vi "DN4_2Darray2DDT.vi"(3 "rate":dbl, 4 "StartTime":timestamp, 5 "2D Array":dbl[][](array[numeric])) -> (1 "Dynamic Data Type":dynamicdata(graph), 2 "EndTime":timestamp)   [LabVIEW 2009]
uses:
  Instance           1 19Saved   2Darray2DDT .vi
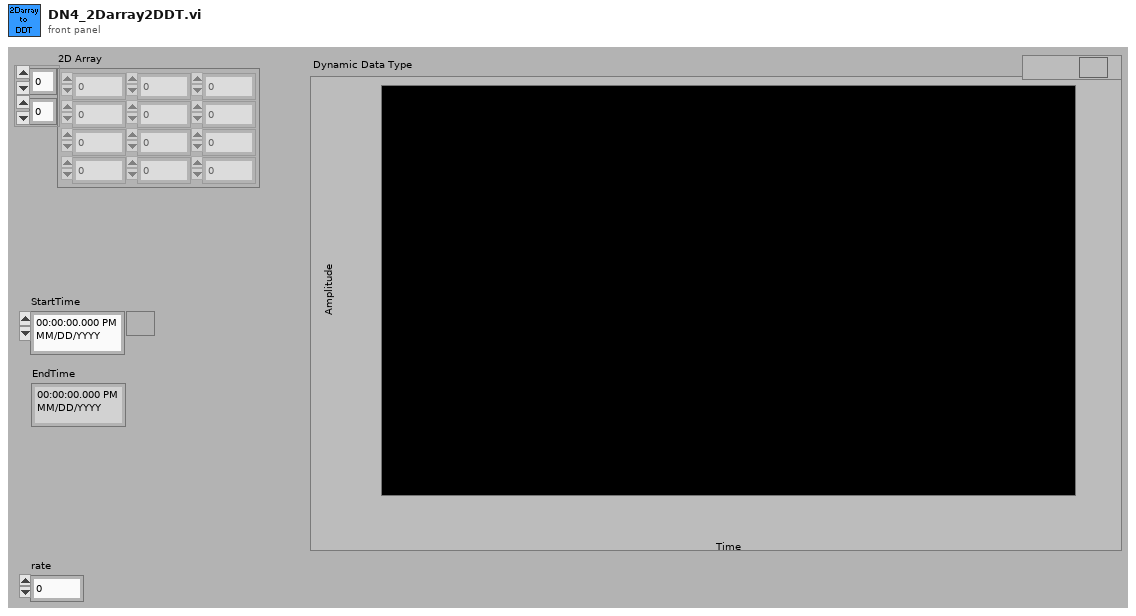
[diagram p1: front panel]
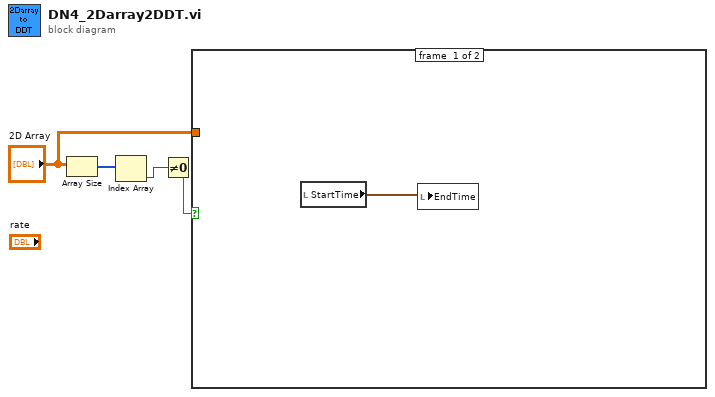
[diagram p0: block diagram]
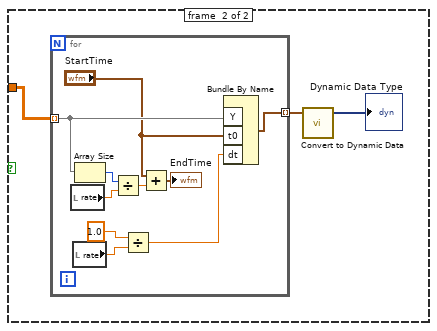
[diagram p2: hidden frame]
diagram:
  n1 = Array Size(array="2D Array") -> (size(s)=w4:i32[])
  n2 = Index Array(array=w4) -> (element=w3:i32)  [unwired: 1 in]
  n3 = Not Equal To 0?(x=w3) -> (x != 0?=w2:bool)
  n4 = case shown="False" w2 {
    tunnel: "2D Array" -> [_ w6]
    frame #0 {
      n5 = local read "StartTime"() -> (w5:timestamp)
      n6 = local write "EndTime"(w5) -> ()
    }
    frame #1 {
      n7 = for {
        tunnel: w6 -> [w16] mode=indexing
        tunnel: [w18] -> w7 mode=indexing
        n8 = local read "rate"() -> (w13:dbl)
        n9 = local read "rate"() -> (w15:dbl)
        n10 = Array Size(array=w16) -> (size(s)=w14:i32)
        n11 = Divide(x=w14, y=w13) -> (x/y=w11:dbl)
        n12 = Divide(x=1.0, y=w15) -> (x/y=w12:dbl)
        n13 = Add(x="StartTime", y=w11) -> (x+y=→"EndTime":timestamp)
        n14 = Bundle By Name("Y"=w16, "t0"="StartTime", "dt"=w12) -> (w18:waveform(dbl))  [unwired: 1 out]
      }
      n15 = call "Convert to Dynamic Data"("Array of Waveforms"=w7) -> ("Dynamic Data Type"=→"Dynamic Data Type":dynamicdata)  [unwired: 3 out]
    }
  }
